vi "current-max-voltage-zero.vi"(6 "Imax (0-3A)":dbl format="%.2f", 7 "error in (no error)":errorcluster, 10 "VISA resource":refnum<visa-resource-name>="PWS4323") -> (0 "error out":errorcluster, 3 "VISA resource name out":refnum<visa-resource-name>)   [LabVIEW 2012]
uses:
  <instrlib>/Tektronix PWS4XXX Series/Tektronix PWS4XXX Series.lvlib
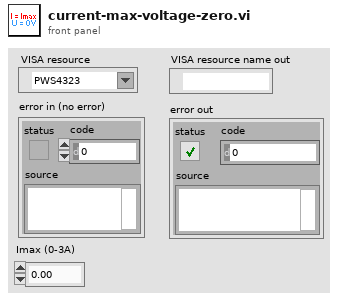
[diagram p1: front panel]
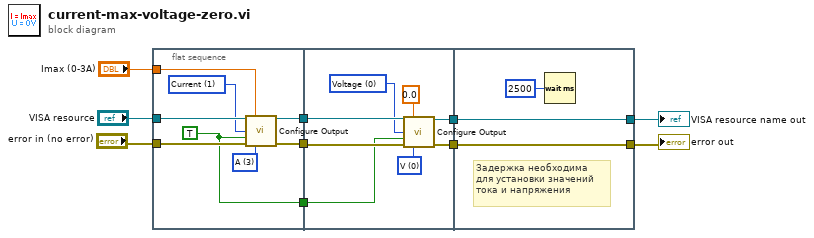
[diagram p0: block diagram]
diagram:
  n1 = flat-sequence {
    tunnel: [w18] -> w10
    tunnel: [w17] -> w9
    tunnel: "error in (no error)" -> [w16]
    tunnel: "VISA resource" -> [w15]
    tunnel: "Imax (0-3A)" -> [w14]
    tunnel: [w11] -> w5
    tunnel: w10 -> [w26]
    tunnel: w9 -> [w25]
    tunnel: w5 -> [w19]
    tunnel: [w21] -> w4
    tunnel: [w20] -> w3
    tunnel: [w28] -> w1
    tunnel: [w29] -> w2
    tunnel: w4 -> [w29]
    tunnel: w3 -> [w28]
    frame #0 {
      w12 = u16 1 items=["Voltage", "Current"] ("Function(0:Voltage)")
      w11 = TRUE ("Enable Output (T: Enable)")
      w13 = u16 3 items=["V", "mV", "kV", "A", "mA"] ("Unit(V)")
      n2 = call <instrlib>:"Configure Output.vi"("VISA resource name"=w15, "Manual Range(0.00)"=w14, "Function(0:Voltage)"=w12, "Enable Output (T: Enable)"=w11, "error in (no error)"=w16, "Unit(V)"=w13) -> ("VISA resource name out"=w18:refnum<visa-resource-name>, "error out"=w17:errorcluster)  [unwired: 8 in]
    }
    frame #1 {
      w22 = u16 0 items=["V", "mV", "kV", "A", "mA"] ("Unit(V)")
      w24 = u16 0 items=["Voltage", "Current"] ("Function(0:Voltage)")
      n3 = call <instrlib>:"Configure Output.vi"("VISA resource name"=w26, "Manual Range(0.00)"=0.0, "Function(0:Voltage)"=w24, "Enable Output (T: Enable)"=w19, "error in (no error)"=w25, "Unit(V)"=w22) -> ("VISA resource name out"=w21:refnum<visa-resource-name>, "error out"=w20:errorcluster)  [unwired: 8 in]
    }
    frame #2 {
      # "Задержка необходима\nдля установки значений\nтока и напряжения"
      n4 = Wait (ms)(milliseconds to wait=u32 2500) -> ()  [unwired: 1 out]
    }
  }
  "VISA resource name out" <- w2
  "error out" <- w1
